vi "Refresh UI Event.vi"(8 "error in (no error)":errorcluster, 11 "Events":T1) -> (0 "error out":errorcluster)   [LabVIEW 2015]
uses:
  TypeDef/EventsReference.ctl
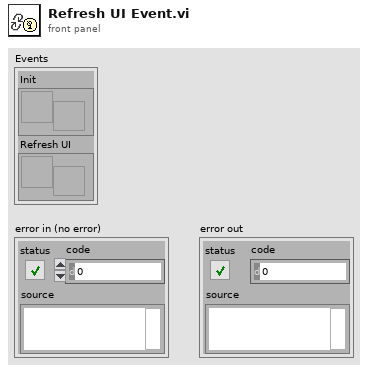
[diagram p1: front panel]
types:
  T1 = typedef "EventsReference.ctl" = cluster{"Init":refnum<user-event>, "Refresh UI":refnum<user-event>}
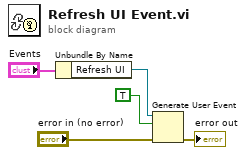
[diagram p0: block diagram]
diagram:
  n1 = Unbundle By Name("Events") -> ("Refresh UI"=w3:refnum<user-event>)
  n2 = Generate User Event(user event=w3, event data cluster=TRUE ("event data"), error in="error in (no error)") -> (error out=→"error out":errorcluster)  [unwired: 1 in, 1 out]
